vi "Read NI 9212.vi"(8 "error in":errorcluster, 11 "NI 9212 in":refnum<class "NI 9212.lvclass">) -> (0 "error out":errorcluster, 1 "module settings":T4={"conversion time"=enum."High Resolution", "open thermocouple detection"=FALSE}, 2 "channel settings":T1[](array[typedef]), 3 "NI 9212 out":refnum<class "NI 9212.lvclass">)   [LabVIEW 2020, in "Scan Engine Scripting.lvlib" / "NI 9212.lvclass"]
doc: "Returns the channel settings of a NI-9212 analog input module that can be edited and then used to create a new module instance to set into a slot."
uses:
  NI 9212.lvclass
  NI 9212 Settings.ctl
  NI 9212 Conversion Time.ctl
  Mode Classes/Controls/thermocouple channel settings.ctl
  Channel Classes/Thermocouple Channel/Thermocouple Type.ctl
  Channel Classes/Thermocouple Channel/Measurement Units.ctl
  Channel Classes/Thermocouple Channel/Thermocouple Channel.lvclass
  Scan Engine Scripting.lvlib
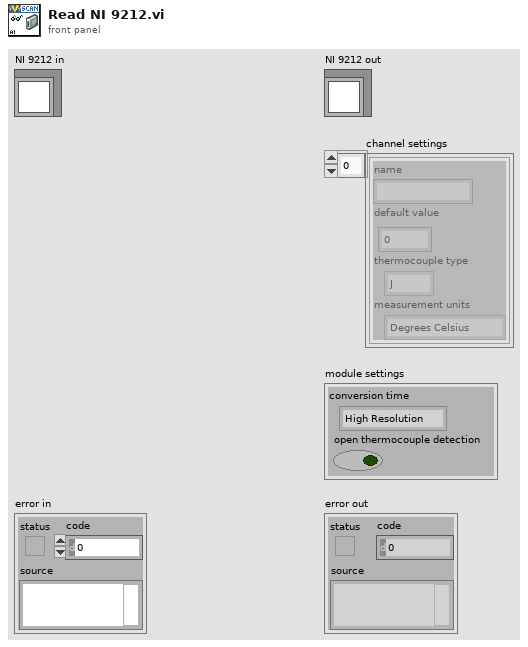
[diagram p1: front panel]
types:
  T1 = typedef "Scan Engine Scripting.lvlib/thermocouple channel settings.ctl" = cluster{"name":string, "default value":dbl, "thermocouple type":T2, "measurement units":T3}
  T2 = typedef "Scan Engine Scripting.lvlib/Thermocouple Channel.lvclass/Thermocouple Type.ctl" = enum16{"J", "K", "T", "E", "R", "S", "N", "B"}
  T3 = typedef "Scan Engine Scripting.lvlib/Thermocouple Channel.lvclass/Measurement Units.ctl" = enum16{"Raw Volts", "Degrees Kelvin", "Degrees Celsius", "Degrees Fahrenheit", "Degrees Rankine"}
  T4 = typedef "Scan Engine Scripting.lvlib/NI 9212.lvclass/NI 9212 Settings.ctl" = cluster{"conversion time":T5, "open thermocouple detection":bool}
  T5 = typedef "Scan Engine Scripting.lvlib/NI 9212.lvclass/NI 9212 Conversion Time.ctl" = enum16{"High Speed", "Best 60 Hz Rejection", "Best 50 Hz Rejection", "High Resolution"}
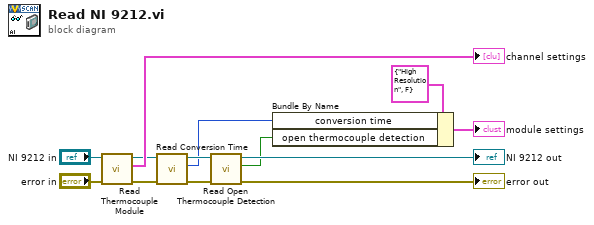
[diagram p0: block diagram]
diagram:
  n1 = call-dynamic "Read Thermocouple Module.vi"("error in"="error in", "module in"="NI 9212 in") -> ("error out"=w10:errorcluster, "channel settings"=→"channel settings":T1[], "module out"=w9:refnum<class "NI 9212.lvclass">)  [unwired: 7 in]
  n2 = call-dynamic "Read Conversion Time.vi"("error in"=w10, "NI 9212 in"=w9) -> ("error out"=w4:errorcluster, "conversion time"=w5:T5, "NI 9212 out"=w8:refnum<class "NI 9212.lvclass">)  [unwired: 7 in]
  n3 = call-dynamic "Read Open Thermocouple Detection.vi"("error in"=w4, "NI 9212 in"=w8) -> ("error out"=→"error out":errorcluster, "open thermocouple detection"=w3:bool, "NI 9212 out"=→"NI 9212 out":refnum<class "NI 9212.lvclass">)  [unwired: 7 in]
  n4 = Bundle By Name(cluster=T4 {"conversion time"=enum."High Resolution", "open thermocouple detection"=FALSE} ("module settings"), "conversion time"=w5, "open thermocouple detection"=w3) -> (→"module settings":T4)
